vi "Will_Waveform_generator.vi"() -> ()   [LabVIEW 2017]
uses:
  <instrlib>/Agilent 33XXX Series/Agilent 33XXX Series.lvlib
panel:
  in  "Delay (0.0 s)":dbl
  in  "Frequency (1000 Hz)":dbl=1000.0
  in  "Amplitude (1)":dbl=1.0
  in  "Waveform Function (1: Sine)":u16(ring)=1 items=["DC", "Sine", "Square", "Triangle", "Ramp", "Pulse", "Noise", "Sinc", "Negative Ramp", "Exponential Rise", "Exponential Fall", "Cardiac"]
  in  "VISA resource name":refnum<visa-resource-name>
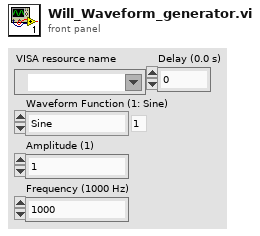
[diagram p1: front panel]
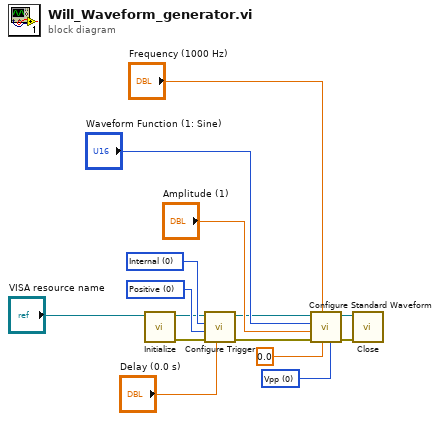
[diagram p0: block diagram]
diagram:
  w6 = u16 0 items=["Positive", "Negative"] ("Slope (0: Positive)")
  w7 = u16 0 items=["Internal", "External", "Software (bus)"] ("Trigger Source (0: Internal)")
  w13 = u16 0 items=["Vpp", "Vrms", "dB"] ("Unit (0: Vpp)")
  n1 = call <instrlib>:"Initialize.vi"("VISA resource name"="VISA resource name") -> ("error out"=w2:errorcluster, "VISA resource name out"=w4:refnum<visa-resource-name>)  [unwired: 9 in]
  n2 = call <instrlib>:"Configure Trigger.vi"("Delay (0.0 s)"="Delay (0.0 s)", "error in (no error)"=w2, "Slope (0: Positive)"=w6, "Trigger Source (0: Internal)"=w7, "VISA resource name"=w4) -> ("error out"=w1:errorcluster, "VISA resource name out"=w3:refnum<visa-resource-name>)  [unwired: 5 in]
  n3 = call <instrlib>:"Configure Standard Waveform.vi"("Unit (0: Vpp)"=w13, "DC Offset (0.00 V)"=0.0, "Frequency (1000 Hz)"="Frequency (1000 Hz)", "error in (no error)"=w1, "Amplitude (1)"="Amplitude (1)", "Waveform Function (1: Sine)"="Waveform Function (1: Sine)", "VISA resource name"=w3) -> ("error out"=w9:errorcluster, "VISA resource name out"=w10:refnum<visa-resource-name>)  [unwired: 3 in]
  n4 = call <instrlib>:"Close.vi"("error in (no error)"=w9, "VISA resource name"=w10) -> ()  [unwired: 9 in, 1 out]
